vi "Write Room Number.vi"(8 "error in (no error)":errorcluster, 10 "Room Number":i32, 11 "Room in":refnum<class "Room.lvclass">) -> (0 "error out":errorcluster, 3 "Room out":refnum<class "Room.lvclass">)   [LabVIEW 2015, in "Room.lvclass"]
uses:
  Room.lvclass
  Room.lvclass/Room.ctl
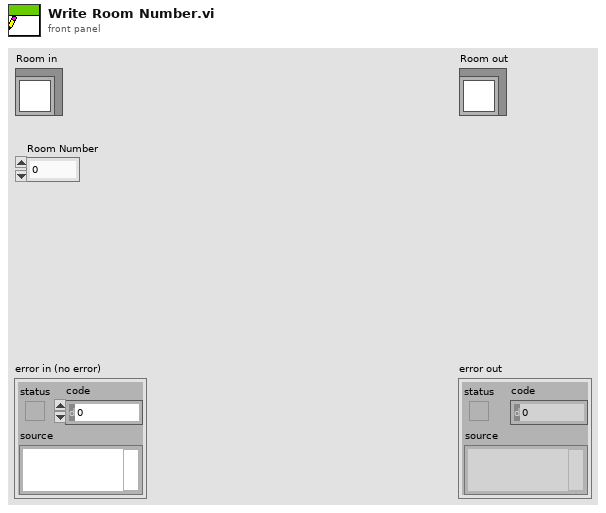
[diagram p1: front panel]
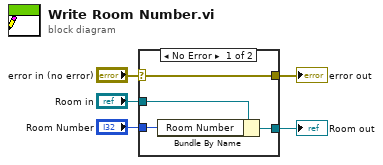
[diagram p0: block diagram]
diagram:
  n1 = case shown="No Error" "error in (no error)" {
    selector: "error in (no error)" -> [w9 w10]
    tunnel: [w9 w10] -> w4
    tunnel: [w7 w11] -> w2
    tunnel: "Room in" -> [w8 w11]
    tunnel: "Room Number" -> [w6 _]
    frame No Error {
      n2 = Bundle By Name(cluster=w8, "Room Number"=w6) -> (w7:refnum<class "Room.lvclass">)
    }
    frame Error {
    }
  }
  "error out" <- w4
  "Room out" <- w2
